vi "Test Instrument Outputs.vi"(8 "error in (no error)":errorcluster, 11 "SR7270 Drivers in":refnum<class "SR7270 Drivers.lvclass">) -> (0 "error out":errorcluster, 3 "SR7270 Drivers out":refnum<class "SR7270 Drivers.lvclass">)   [LabVIEW 2016, in "SR7270 Drivers.lvclass"]
uses:
  SR7270 Drivers.lvclass
  SR7270 Drivers.lvclass/SR7270 Drivers.ctl
  <vilib>/addons/_JKI Toolkits/Caraya/classes/Test/Test.lvclass
  <vilib>/addons/_JKI Toolkits/Caraya/classes/Assert/Assert.lvclass
panel:
  out "time (ms)":u32
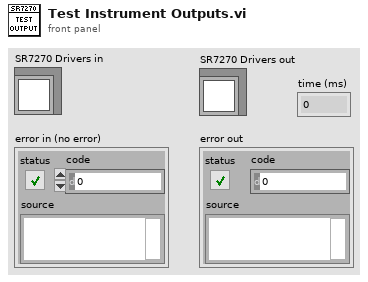
[diagram p1: front panel]
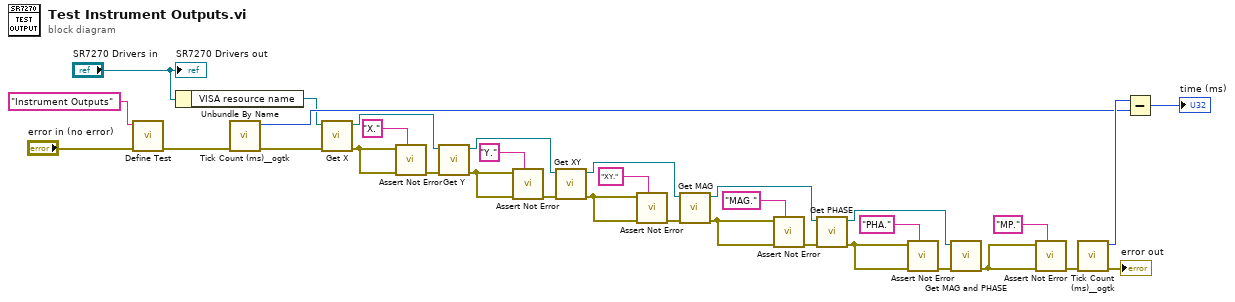
[diagram p0: block diagram]
diagram:
  n1 = call <vilib>:"Define Test.vi"("error in (no error)"="error in (no error)", "Label (VI Title)"="Instrument Outputs") -> ("error out"=w31:errorcluster)  [unwired: 9 in]
  n2 = Unbundle By Name("SR7270 Drivers in") -> ("VISA resource name"=w2:refnum<visa-resource-name>)
  n3 = call <userlib>:"Tick Count (ms)__ogtk.vi"("error in (no error)"=w31) -> ("error out"=w7:errorcluster, "millisecond timer value"=w4:u32)  [unwired: 9 in]
  n4 = call "Get X.vi"("error in (no error)"=w7, "VISA resource name"=w2) -> ("error out"=w18:errorcluster, "VISA resource name out"=w30:refnum<visa-resource-name>)  [unwired: 7 in, 1 out]
  n5 = call <vilib>:"Assert Not Error.vi"("Label"="X.", "error in (no error)"=w18, "Not Error?"=w18) -> ("error out"=w23:errorcluster)  [unwired: 8 in]
  n6 = call "Get Y.vi"("error in (no error)"=w23, "VISA resource name"=w30) -> ("error out"=w17:errorcluster, "VISA resource name out"=w29:refnum<visa-resource-name>)  [unwired: 7 in, 1 out]
  n7 = call <vilib>:"Assert Not Error.vi"("Label"="Y.", "error in (no error)"=w17, "Not Error?"=w17) -> ("error out"=w22:errorcluster)  [unwired: 8 in]
  n8 = call "Get XY.vi"("error in (no error)"=w22, "VISA resource name"=w29) -> ("error out"=w16:errorcluster, "VISA resource name out"=w28:refnum<visa-resource-name>)  [unwired: 6 in, 2 out]
  n9 = call <vilib>:"Assert Not Error.vi"("Label"="XY.", "error in (no error)"=w16, "Not Error?"=w16) -> ("error out"=w21:errorcluster)  [unwired: 8 in]
  n10 = call "Get MAG.vi"("error in (no error)"=w21, "VISA resource name"=w28) -> ("error out"=w15:errorcluster, "VISA resource name out"=w27:refnum<visa-resource-name>)  [unwired: 7 in, 1 out]
  n11 = call <vilib>:"Assert Not Error.vi"("Label"="MAG.", "error in (no error)"=w15, "Not Error?"=w15) -> ("error out"=w20:errorcluster)  [unwired: 8 in]
  n12 = call "Get PHASE.vi"("error in (no error)"=w20, "VISA resource name"=w27) -> ("error out"=w14:errorcluster, "VISA resource name out"=w26:refnum<visa-resource-name>)  [unwired: 7 in, 1 out]
  n13 = call <vilib>:"Assert Not Error.vi"("Label"="PHA.", "error in (no error)"=w14, "Not Error?"=w14) -> ("error out"=w19:errorcluster)  [unwired: 8 in]
  n14 = call "Get MAG and PHASE.vi"("error in (no error)"=w19, "VISA resource name"=w26) -> ("error out"=w25:errorcluster)  [unwired: 6 in, 3 out]
  n15 = call <vilib>:"Assert Not Error.vi"("Label"="MP.", "error in (no error)"=w25, "Not Error?"=w25) -> ("error out"=w24:errorcluster)  [unwired: 8 in]
  n16 = call <userlib>:"Tick Count (ms)__ogtk.vi"("error in (no error)"=w24) -> ("error out"=→"error out":errorcluster, "millisecond timer value"=w5:u32)  [unwired: 9 in]
  n17 = Subtract(x=w5, y=w4) -> (x-y=→"time (ms)":u32)
  "SR7270 Drivers out" <- "SR7270 Drivers in"
